vi "Write-Read TPI Demo.vi"(5 "Write Buffer":u8[](array[numeric])=[170, 85, 0, 2, 8, 1, 244] format="%x", 6 "Device Index":u32=1) -> (0 "Bytes Read":u32, 3 "Read Buffer Out":u8[](array[numeric])=[170, 85, 0, 2, 8, 1, 244] format="%x", 4 "Bytes Written":u32=7)   [LabVIEW 2013]
panel:
  in  "Flow Control":u16(ring)=256 items=["None"=0, "RTS-CTS"=256, "DTR-DSR"=512, "XOn-XOff"=1024]
  in  "Parity":u8(ring) items=["FT_PARITY_NONE", "FT_PARITY_ODD", "FT_PARITY_EVEN", "FT_PARITY_MARK", "FT_PARITY_SPACE"]
  in  "Stop Bits":u8(ring) items=["FT_STOP_BITS_1"=0, "FT_STOP_BITS_2"=2]
  in  "Word Length":u8(ring)=8 items=["FT_BITS_7"=7, "FT_BITS_8"=8]
  in  "Baud Rate":u32=3000000
  out "Device Description":string="FT230X Basic UART"
  out "Bytes Waiting":u32
  # "Enter values in Write Buffer and run program.  \nWith a loop-back connector, the data is read back into the Read Buffer."
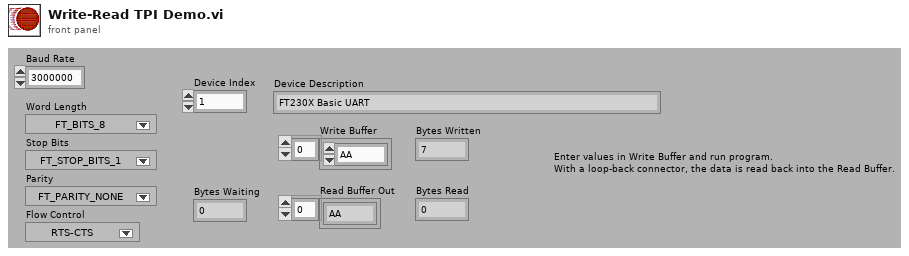
[diagram p1: front panel]
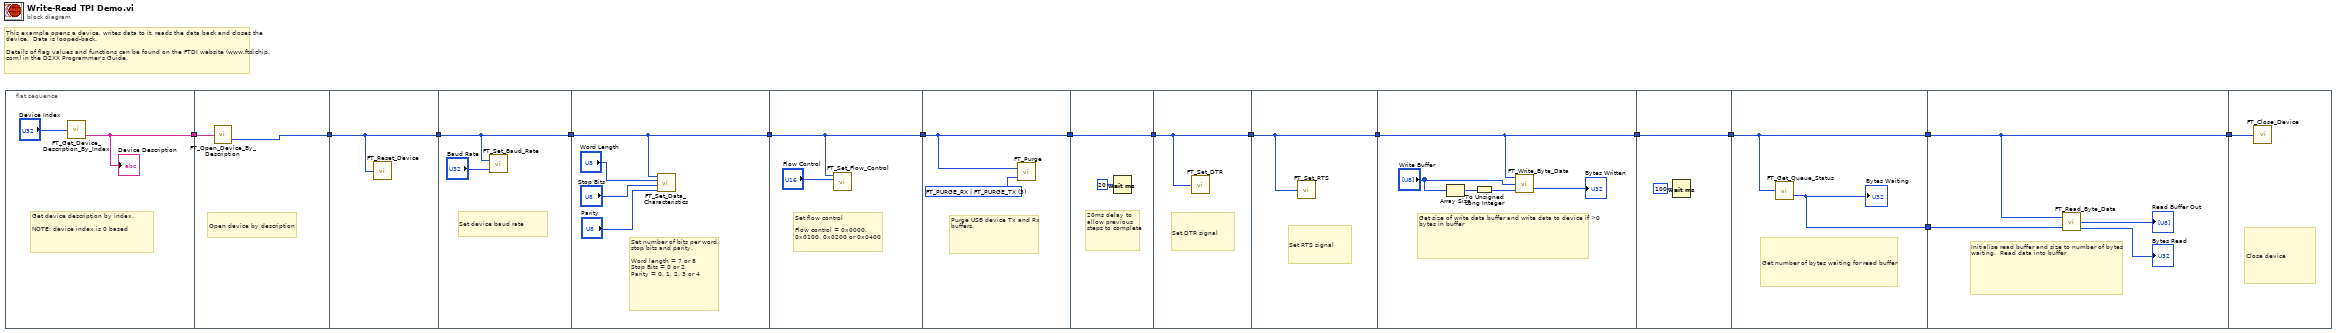
[diagram p0: block diagram]
diagram:
  # "This example opens a device, writes data to it, reads the data back and closes the device.  Data is looped-back.\n\nDetails of flag values and functions can be found on the FTDI website (www.ftdichip.com) in the D2XX Programmer's Guide."
  n1 = flat-sequence {
    tunnel: [w17] -> w11
    tunnel: [w19] -> w9
    tunnel: w11 -> [w18]
    tunnel: w9 -> [w20]
    tunnel: [w20] -> w8
    tunnel: w8 -> [w21]
    tunnel: [w21] -> w3
    tunnel: w3 -> [w26]
    tunnel: [w26] -> w15
    tunnel: w15 -> [w28]
    tunnel: [w28] -> w2
    tunnel: w2 -> [w30]
    tunnel: [w30] -> w1
    tunnel: [w31] -> w10
    tunnel: w1 -> [w31]
    tunnel: w10 -> [w33]
    tunnel: [w33] -> w7
    tunnel: w7 -> [w34]
    tunnel: [w34] -> w6
    tunnel: w6 -> [w39]
    tunnel: [w39] -> w5
    tunnel: w5 -> [w41]
    tunnel: [w41] -> w14
    tunnel: w14 -> [w43]
    tunnel: [w43] -> w13
    tunnel: [w42] -> w12
    tunnel: w13 -> [w46]
    tunnel: [w46] -> w4
    tunnel: w12 -> [w44]
    tunnel: w4 -> [w48]
    frame #0 {
      # "Get device description by index.\n\nNOTE: device index is 0 based"
      n2 = call "FT_Get_Device_Description_By_Index.vi"("Device Index"="Device Index") -> ("Device Description"=w17:string)  [unwired: 1 out]
      "Device Description" <- w17
    }
    frame #1 {
      # "Open device by description"
      n3 = call "FT_Open_Device_By_Description.vi"("Device Description"=w18) -> ("Handle"=w19:u32)  [unwired: 1 out]
    }
    frame #2 {
      n4 = call "FT_Reset_Device.vi"("Handle"=w20) -> ()  [unwired: 1 out]
    }
    frame #3 {
      # "Set device baud rate"
      n5 = call "FT_Set_Baud_Rate.vi"("Baud Rate"="Baud Rate", "Handle"=w21) -> ()  [unwired: 1 out]
    }
    frame #4 {
      # "Set number of bits per word, stop bits and parity.\n\nWord length = 7 or 8\nStop Bits = 0 or 2\nParity = 0, 1, 2, 3 or 4"
      n6 = call "FT_Set_Data_Characteristics.vi"("Parity"="Parity", "Stop Bits"="Stop Bits", "Word Length"="Word Length", "Handle"=w26) -> ()  [unwired: 1 out]
    }
    frame #5 {
      # "Set flow control\n\nFlow control = 0x0000, 0x0100, 0x0200 or 0x0400"
      n7 = call "FT_Set_Flow_Control.vi"("Flow Control"="Flow Control", "Handle"=w28) -> ()  [unwired: 2 in, 1 out]
    }
    frame #6 {
      w29 = u32 3 items=["FT_PURGE_RX"=1, "FT_PURGE_TX"=2, "FT_PURGE_RX | FT_PURGE_TX"=3] ("Purge Flags")
      # "Purge USB device Tx and Rx  buffers."
      n8 = call "FT_Purge.vi"("Purge Flags"=w29, "Handle"=w30) -> ()  [unwired: 1 out]
    }
    frame #7 {
      # "20ms delay to allow previous steps to complete"
      n9 = Wait (ms)(milliseconds to wait=u32 20) -> ()  [unwired: 1 out]
    }
    frame #8 {
      # "Set DTR signal"
      n10 = call "FT_Set_DTR.vi"("Handle"=w33) -> ()  [unwired: 1 out]
    }
    frame #9 {
      # "Set RTS signal"
      n11 = call "FT_Set_RTS.vi"("Handle"=w34) -> ()  [unwired: 1 out]
    }
    frame #10 {
      # "Get size of write data buffer and write data to device if >0 bytes in buffer"
      n12 = Array Size(array="Write Buffer") -> (size(s)=w35:i32)
      n13 = To Unsigned Long Integer(number=w35) -> (unsigned 32bit integer=w36:u32)
      n14 = call "FT_Write_Byte_Data.vi"("Bytes To Write"=w36, "Buffer"="Write Buffer", "Handle"=w39) -> ("Bytes Written"=→"Bytes Written":u32)  [unwired: 1 out]
    }
    frame #11 {
      n15 = Wait (ms)(milliseconds to wait=u32 100) -> ()  [unwired: 1 out]
    }
    frame #12 {
      # "Get number of bytes waiting for read buffer"
      n16 = call "FT_Get_Queue_Status.vi"("Handle"=w43) -> ("Bytes Waiting"=w42:u32)  [unwired: 1 out]
      "Bytes Waiting" <- w42
    }
    frame #13 {
      # "Initialise read buffer and size to number of bytes waiting.  Read data into buffer"
      n17 = call "FT_Read_Byte_Data.vi"("Handle"=w46, "Bytes To Read"=w44) -> ("Read Data"=→"Read Buffer Out":u8[], "Bytes Read"=→"Bytes Read":u32)  [unwired: 1 out]
    }
    frame #14 {
      # "Close device"
      n18 = call "FT_Close_Device.vi"("Handle"=w48) -> ()  [unwired: 1 out]
    }
  }
